vi "CurrentSetZ.vi"(8 "error in (no error)":errorcluster, 10 "Cluster":T1={"VISA resource name"="COM6", "baud rate (9600)"=9600, "data bits (8)"=8, "parity (0:none)"=enum."None"} {"data bits (8)" min=5 max=8 step=1}, 11 "电流设置":dbl min=-5.0 max=5.0 step=0.2) -> (0 "error out":errorcluster)   [LabVIEW 2020, in "YP03-60CurrentSource_1.lvlib"]
uses:
  Libraries/YP03-60CurrentSource_1/YP03-60CurrentSource_1.lvlib
  <vilib>/Instr/_visa.llb/VISA Configure Serial Port (Instr).vi
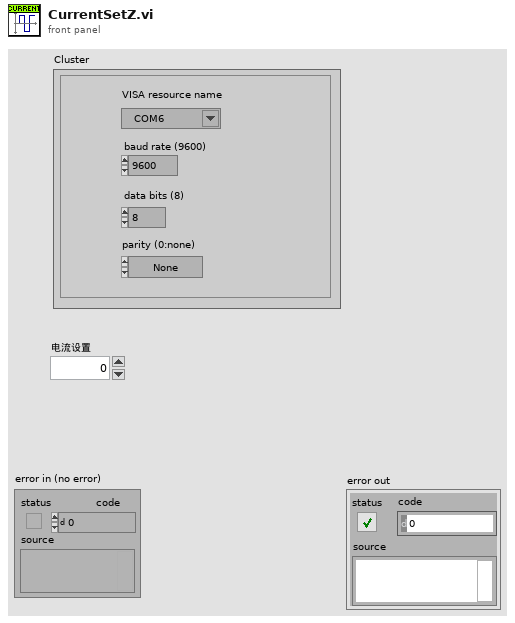
[diagram p1: front panel]
types:
  T1 = cluster{"VISA resource name":refnum<visa-resource-name>, "baud rate (9600)":u32, "data bits (8)":u16, "parity (0:none)":enum16{"None", "Odd", "Even", "Mark", "Space"}}
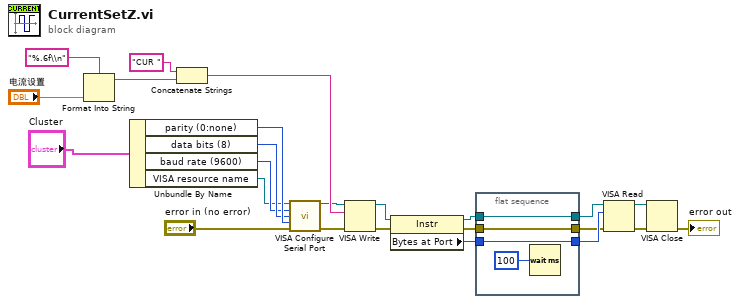
[diagram p0: block diagram]
diagram:
  n1 = Format Into String(format string="%.6f\\n", "电流设置") -> (resulting string=w17:string)  [unwired: 2 in, 1 out]
  n2 = Unbundle By Name("Cluster") -> ("parity (0:none)"=w24:enum16{"None", "Odd", "Even", "Mark", "Space"}, "data bits (8)"=w23:u16, "baud rate (9600)"=w22:u32, "VISA resource name"=w21:refnum<visa-resource-name>)
  n3 = Concatenate Strings("CUR " ("string"), w17) -> (w13:string)
  n4 = call-poly "VISA Configure Serial Port"("VISA resource name"=w21, "baud rate (9600)"=w22, "data bits (8)"=w23, "parity (0:none)"=w24, "error in (no error)"="error in (no error)") -> ("VISA resource name out"=w6:refnum<visa-resource-name>, "error out"=w5:errorcluster)  [unwired: 9 in]
  n5 = VISA Write(VISA resource name=w6, write buffer=w13, error in (no error)=w5) -> (VISA resource name out=w15:refnum<visa-resource-name>, error out=w14:errorcluster)  [unwired: 1 out]
  n6 = property class="Instr"(reference=w15, error in=w14) -> (reference out=w10:refnum<visa-resource-name>, error out=w8:errorcluster, "Bytes at Port"=w12:u32)
  n7 = flat-sequence {
    tunnel: w10 -> [w28]
    tunnel: [w28] -> w9
    tunnel: [w27] -> w7
    tunnel: w8 -> [w27]
    tunnel: [w26] -> w11
    tunnel: w12 -> [w26]
    frame #0 {
      n8 = Wait (ms)(milliseconds to wait=u32 100) -> ()  [unwired: 1 out]
    }
  }
  n9 = VISA Read(VISA resource name=w9, byte count=w11, error in (no error)=w7) -> (VISA resource name out=w2:refnum<visa-resource-name>, error out=w3:errorcluster)  [unwired: 2 out]
  n10 = VISA Close(VISA resource name=w2, error in (no error)=w3) -> (error out=→"error out":errorcluster)
